vi "Apply Profile to Repeated Pattern.vi"(0 "profile array":dbl[](array[numeric]), 5 "pattern":dbl[](array[numeric]), 7 "alignment":enum16{"Beginning", "End"}(ring)) -> (4 "profiled pattern":dbl[](array[numeric]))   [LabVIEW 2017, in "SV Signal.lvclass"]
uses:
  <vilib>/addons/_NISVFA/_Generation/Signal Generation/SV Signal/SV Signal.lvclass
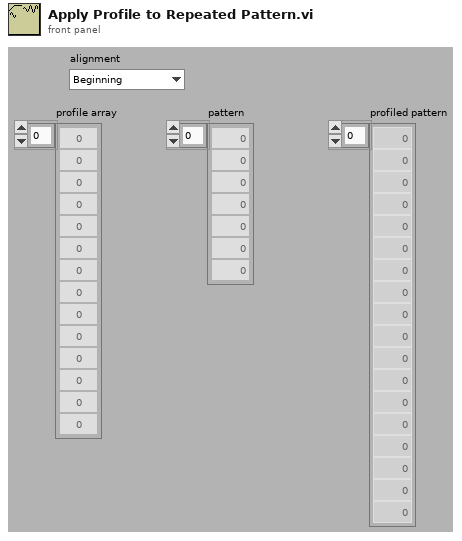
[diagram p1: front panel]
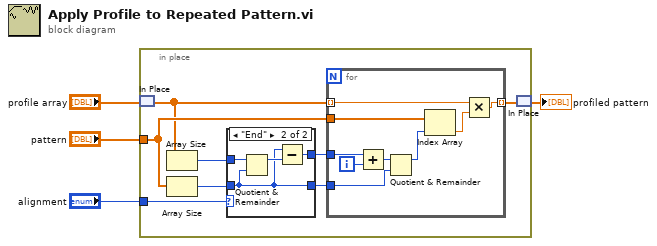
[diagram p0: block diagram]
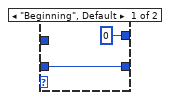
[diagram p2: hidden frame]
diagram:
  n1 = in-place {
    in-place-border: "alignment" -> [w9]
    in-place-border: "pattern" -> [w8]
    n2 = in-place-match #1("profile array") -> (w7:dbl[])
    n3 = Array Size(array=w7) -> (size(s)=w12:i32)
    n4 = Array Size(array=w8) -> (size(s)=w10:i32)
    n5 = case shown="\"End\"" w9 {
      tunnel: w12 -> [_ w18]
      tunnel: [0 w16] -> w11
      tunnel: w10 -> [w13 w15]
      tunnel: [w13 w15] -> w5
      frame "Beginning", Default {
      }
      frame "End" {
        n6 = Quotient & Remainder(x=w18, y=w15) -> (x-y*floor(x/y)=w17:i32)  [unwired: 1 out]
        n7 = Subtract(x=w15, y=w17) -> (x-y=w16:i32)
      }
    }
    n8 = for {
      tunnel: w7 -> [w24] mode=indexing
      tunnel: w8 -> [w27]
      tunnel: w11 -> [w26]
      tunnel: [w22] -> w6 mode=indexing
      tunnel: w5 -> [w19]
      i -> [w25]
      n9 = Add(x=w26, y=w25) -> (x+y=w21:i32)
      n10 = Quotient & Remainder(x=w21, y=w19) -> (x-y*floor(x/y)=w20:i32)  [unwired: 1 out]
      n11 = Index Array(array=w27, index=w20) -> (element=w23:dbl)
      n12 = Multiply(x=w24, y=w23) -> (x*y=w22:dbl)
    }
    n13 = in-place-match #1(w6) -> (→"profiled pattern":dbl[])
  }
